vi "tiwi-5-final.vi"() -> ()   [LabVIEW 2013]
panel:
  out "STOP led":bool
  out "Waveform Graph 2":dbl[](graph)
  out "Waveform Graph":dbl[](graph)
  out "Waveform Chart":dbl(graph)
  out "number (0 to 1)":dbl
  in  "Stop":bool
  out "Current Data Value":dbl
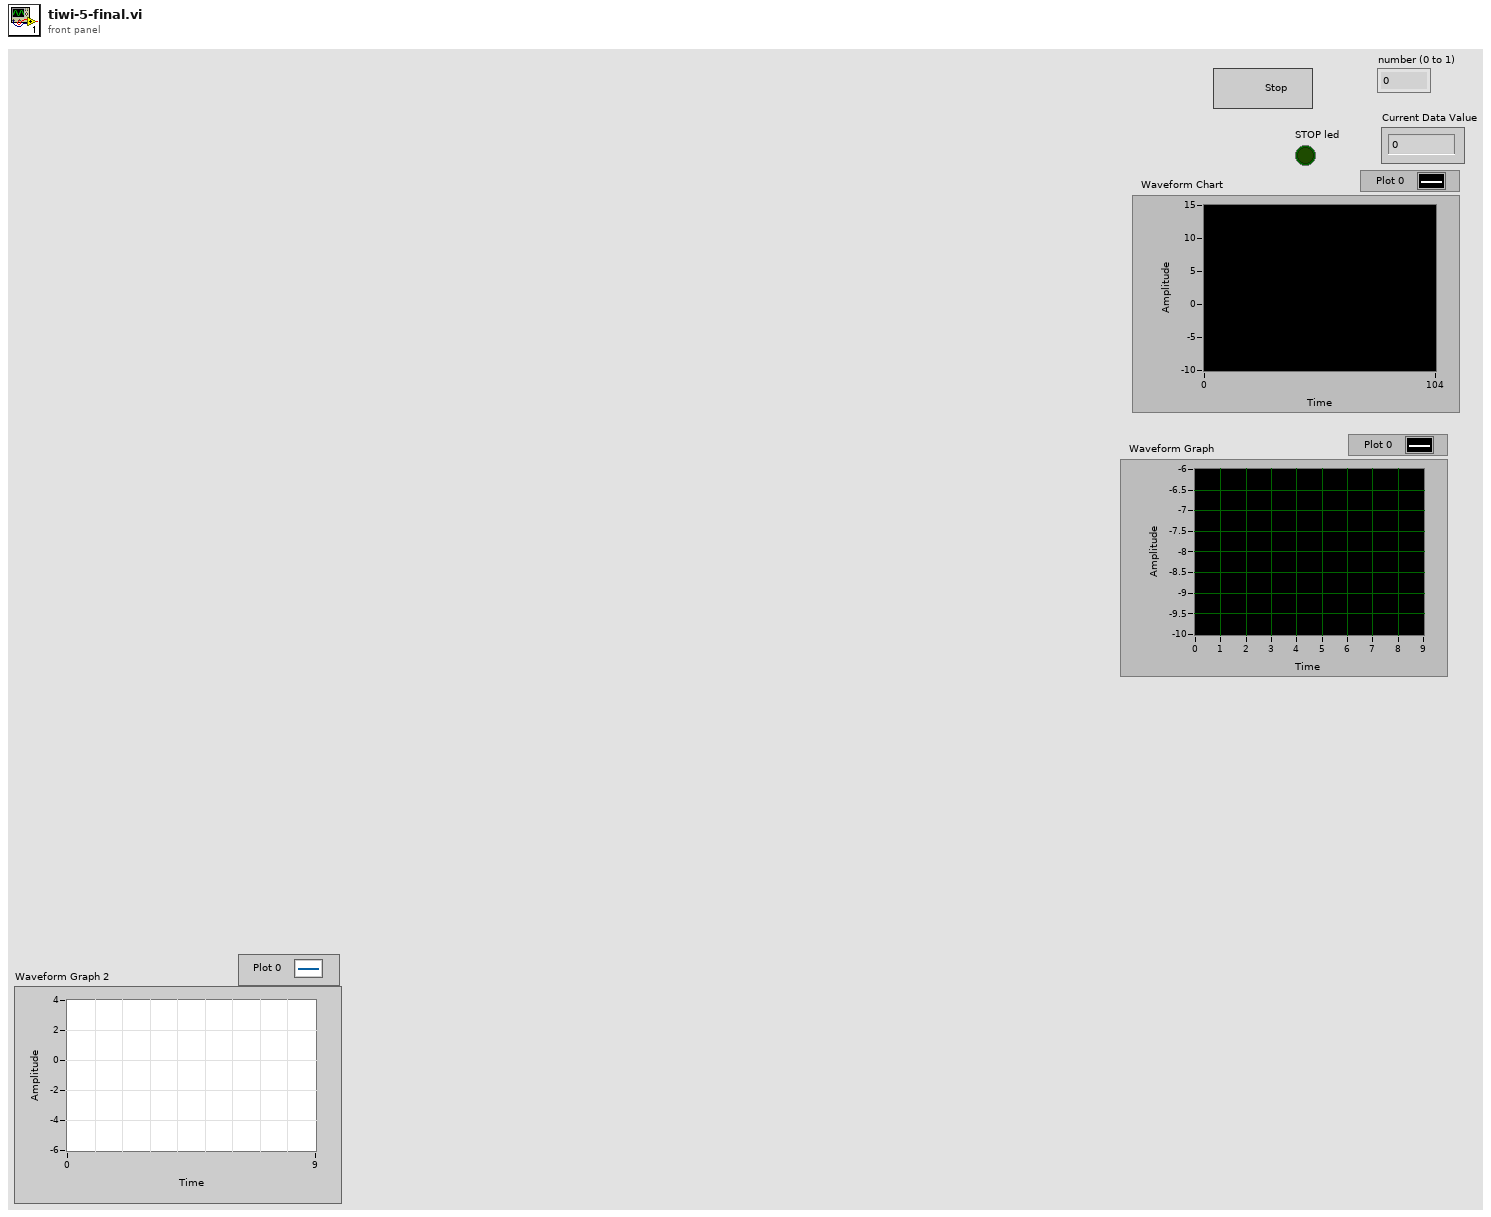
[diagram p1: front panel]
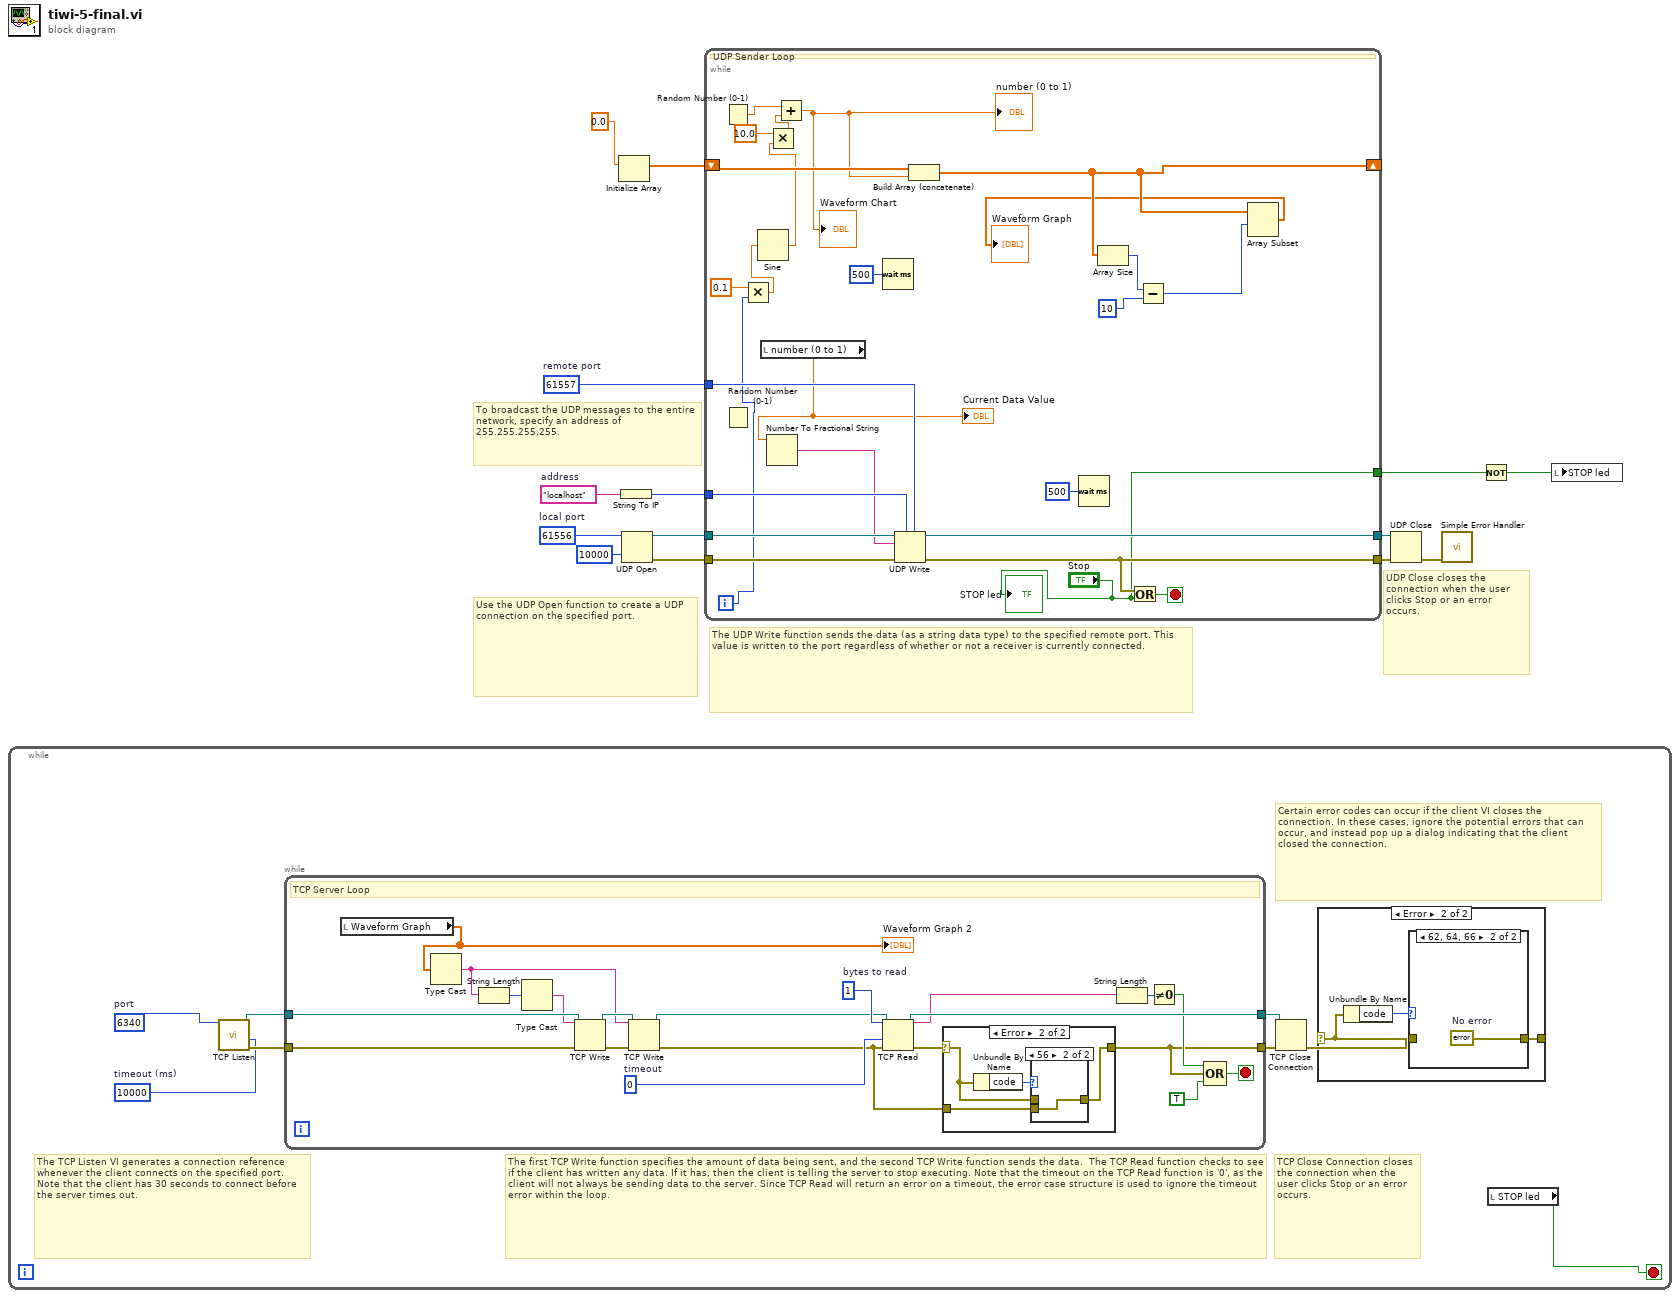
[diagram p0: block diagram]
diagram:
  w5 = u16 61557  # remote port
  w6 = u16 61556  # local port
  w11 = "localhost"  # address
  # "To broadcast the UDP messages to the entire network, specify an address of 255.255.255.255."
  # "UDP Close closes the connection when the user clicks Stop or an error occurs."
  # "The UDP Write function sends the data (as a string data type) to the specified remote port. This value is written to the port regardless of whether or not a receiver is currently connected."
  # "Use the UDP Open function to create a UDP connection on the specified port."
  n1 = while {
    stop <- w15 stop-if-true
    w16 = u16 6340  # port
    w17 = 10000  # timeout (ms)
    # "TCP Close Connection closes the connection when the user clicks Stop or an error occurs."
    # "The TCP Listen VI generates a connection reference whenever the client connects on the specified port. Note that the client has 30 seconds to connect before the server times out."
    # "Certain error codes can occur if the client VI closes the connection. In these cases, ignore the potential errors that can occur, and instead pop up a dialog indicating that the client closed the connection."
    # "The first TCP Write function specifies the amount of data being sent, and the second TCP Write function sends the data.  The TCP Read function checks to see if the client has written any data. If it has, then the client is telling the server to stop executing. Note that the timeout on the TCP Read function is '0', as the client will not always be sending data to the server. Since TCP Read will return an error on a timeout, the error case structure is used to ignore the timeout error within the loop."
    n2 = call <vilib>:"TCP Listen.vi"("timeout ms (wait forever: -1)"=w17, "port"=w16) -> ("error out"=w18:errorcluster, "connection ID"=w19:refnum<k5>)  [unwired: 5 in, 3 out]
    n3 = while {
      tunnel: [w33] -> w21
      tunnel: [w39] -> w22
      tunnel: w19 -> [w48]
      tunnel: w18 -> [w41]
      stop <- w42 stop-if-true
      w38 = 0  # timeout
      w40 = 1  # bytes to read
      # "TCP Server Loop"
      n4 = local read "Waveform Graph"() -> (w30:dbl[])
      "Waveform Graph 2" <- w30
      n5 = Type Cast(x=w30) -> (*(type *) &x=w43:string)  [unwired: 1 out]
      n6 = String Length(string=w43) -> (length=w45:i32)
      n7 = Type Cast(x=w45) -> (*(type *) &x=w44:string)  [unwired: 1 out]
      n8 = TCP Write(connection ID=w48, data in=w44, error in (no error)=w41) -> (connection ID out=w47:refnum<k5>, error out=w46:errorcluster)  [unwired: 2 out]
      n9 = TCP Write(connection ID=w47, data in=w43, error in (no error)=w46) -> (connection ID out=w32:refnum<k5>, error out=w31:errorcluster)  [unwired: 2 out]
      n10 = TCP Read(connection ID=w32, bytes to read=w40, error in (no error)=w31, 9:w38) -> (connection ID out=w39:refnum<k5>, data out=w36:string, error out=w34:errorcluster)  [unwired: 1 out]
      n11 = case shown="Error" w34 {
        selector: w34 -> [w49 w52]
        tunnel: [w49 w50] -> w33
        tunnel: w31 -> [_ w51]
        frame No Error {
        }
        frame Error {
          n12 = Unbundle By Name(w52) -> ("code"=w53:i32)
          n13 = case shown="56" w53 {
            tunnel: w52 -> [w54 _]
            tunnel: w51 -> [_ w55]
            tunnel: [w54 w55] -> w50
            frame Default {
            }
            frame 56 {
            }
          }
        }
      }
      n14 = String Length(string=w36) -> (length=w37:i32)
      n15 = Not Equal To 0?(x=w37) -> (x != 0?=w35:bool)
      n16 = Compound Arithmetic op=OR(w35, w33, TRUE) -> (w42:bool)
    }
    n17 = TCP Close Connection(connection ID=w22, error in (no error)=w21) -> (error out=w20:errorcluster)  [unwired: 2 out]
    n18 = case shown="Error" w20 {
      selector: w20 -> [w23 w25]
      tunnel: [w23 w24] -> _
      frame No Error {
      }
      frame Error {
        n19 = Unbundle By Name(w25) -> ("code"=w26:i32)
        n20 = case shown="62, 64, 66" w26 {
          tunnel: w25 -> [w27 _]
          tunnel: [w27 w28] -> w24
          frame Default {
          }
          frame 62, 64, 66 {
            w28 = errorcluster {"status"=FALSE, "code"=0, "source"=""}  # No error
          }
        }
      }
    }
    n21 = local read "STOP led"() -> (w15:bool)
  }
  n22 = Initialize Array(0.0 ("element")) -> (w4:dbl[])  [unwired: 1 in]
  n23 = String To IP(1:w11) -> (0:w9:u32)
  n24 = UDP Open(9:10000 ("timeout ms (25000)"), 11:w6) -> (port=w8:refnum<k16>, 0:w7:errorcluster)  [unwired: 3 in, 1 out]
  n25 = while {
    tunnel: [w77] -> w12
    tunnel: w8 -> [w81]
    tunnel: w7 -> [w80]
    tunnel: [w78] -> w13
    tunnel: w9 -> [w76]
    tunnel: w5 -> [w73]
    shift-right: [w67] -> _
    shift-left: w4 -> [w71]
    tunnel: ["Stop"] -> w3
    i -> [w62]
    stop <- w79 stop-if-true
    # "UDP Sender Loop"
    n26 = Random Number (0-1)() -> (number: 0 to 1=w58:dbl)
    n27 = Random Number (0-1)() -> ()  [unwired: 1 out]
    n28 = Multiply(x=0.1, y=w62) -> (x*y=w61:dbl)
    n29 = Sine(x=w61) -> (sin(x)=w60:dbl)
    n30 = local read "number (0 to 1)"() -> (w70:dbl)
    "Current Data Value" <- w70
    n31 = Number To Fractional String(number=w70) -> (F-format string=w74:string)  [unwired: 3 in]
    n32 = Multiply(x=10.0, y=w60) -> (x*y=w57:dbl)
    n33 = Add(x=w58, y=w57) -> (x+y=w56:dbl)
    "number (0 to 1)" <- w56
    "Waveform Chart" <- w56
    n34 = Wait (ms)(milliseconds to wait=u32 500) -> ()  [unwired: 1 out]
    n35 = UDP Write(address=w76, port or service name=w73, connection ID=w81, data in=w74, 8:w80) -> (error out=w77:errorcluster, 3:w78:refnum<k16>)  [unwired: 1 in]
    n36 = Build Array (concatenate)(w71, w56) -> (w67:dbl[])
    n37 = Wait (ms)(milliseconds to wait=u32 500) -> ()  [unwired: 1 out]
    n38 = Array Size(array=w67) -> (size(s)=w68:i32)
    n39 = Or(x=w77, y="Stop") -> (x .or. y?=w79:bool)
    n40 = Subtract(x=w68, y=10 ("x")) -> (x-y=w66:i32)
    n41 = Array Subset(array=w67, index=w66) -> (→"Waveform Graph":dbl[])  [unwired: 1 in]
    "STOP led" <- "Stop"
  }
  n42 = UDP Close(connection ID=w13, 8:w12) -> (error out=w10:errorcluster)  [unwired: 1 out]
  n43 = call <vilib>:"Simple Error Handler.vi"("error in (no error)"=w10) -> ()  [unwired: 4 in, 5 out]
  n44 = Not(x=w3) -> (.not. x?=w2:bool)
  n45 = local write "STOP led"(w2) -> ()
